vi "part_2.vi"() -> ()   [LabVIEW 2023]
panel:
  in  "check":bool
  in  "stop":bool
  in  "stop 2":bool
  out "Array":bool[](array[boolean])
  in  "Enum":enum16{"XOr", "Or", "And"}(ring)
  out "Boolean 24":bool
  out "Boolean 23":bool
  out "Boolean 22":bool
  out "Boolean 21":bool
  out "Boolean 20":bool
  out "Boolean 19":bool
  out "Boolean 18":bool
  out "Boolean 17":bool
  in  "Boolean 16":bool
  in  "Boolean 15":bool
  in  "Boolean 14":bool
  in  "Boolean 13":bool
  in  "Boolean 12":bool
  in  "Boolean 11":bool
  in  "Boolean 10":bool
  in  "Boolean 9":bool
  in  "Boolean 8":bool
  in  "Boolean 7":bool
  in  "Boolean 6":bool
  in  "Boolean 5":bool
  in  "Boolean 4":bool
  in  "Boolean 3":bool
  in  "Boolean 2":bool
  in  "Boolean":bool
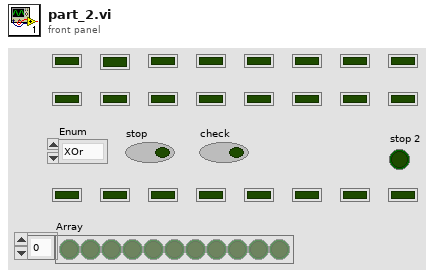
[diagram p1: front panel]
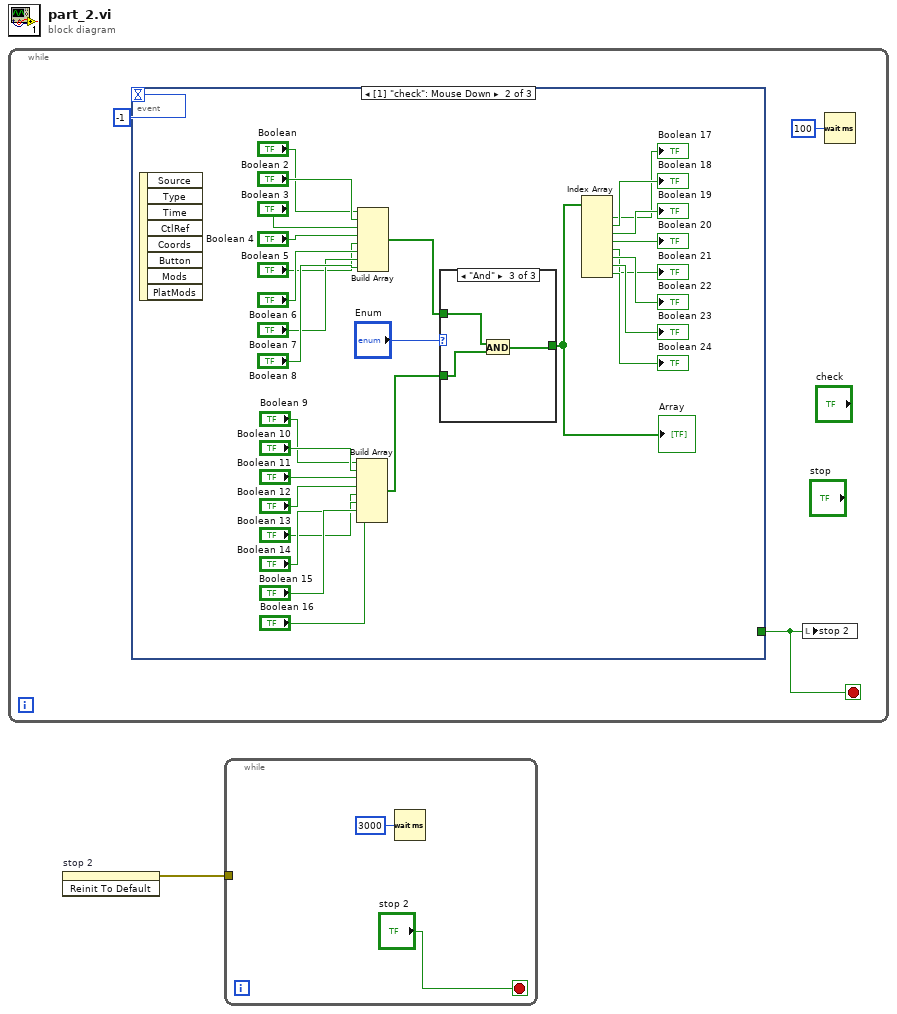
[diagram p0: block diagram]
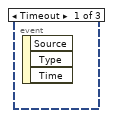
[diagram p2: hidden frame]
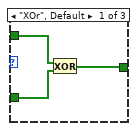
[diagram p3: hidden frame]
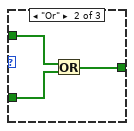
[diagram p4: hidden frame]
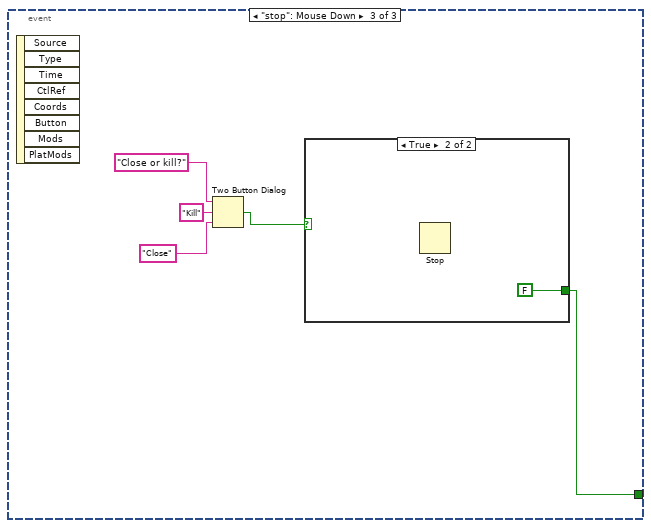
[diagram p5: hidden frame]
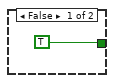
[diagram p6: hidden frame]
diagram:
  n1 = while {
    stop <- w3 stop-if-true
    n2 = event shown="[1] \"check\": Mouse Down" {
      selector: _ -> [_ _ _]
      dyn-events: _ -> [_ _ _]
      timeout: -1 -> [_ _ _]
      tunnel: [_ _ w42] -> w3
      event Timeout {
        n3 = event-data() -> ()  [unwired: 1 in, 3 out]
      }
      event "check": Mouse Down {
        n4 = event-data() -> ()  [unwired: 1 in, 8 out]
        n5 = Build Array("Boolean 9", "Boolean 10", "Boolean 11", "Boolean 12", "Boolean 13", "Boolean 14", "Boolean 15", "Boolean 16") -> (w23:bool[])
        n6 = Build Array("Boolean", "Boolean 2", "Boolean 3", "Boolean 4", "Boolean 5", "Boolean 6", "Boolean 7", "Boolean 8") -> (w22:bool[])
        n7 = case shown="\"And\"" "Enum" {
          tunnel: w22 -> [w33 w37 w40]
          tunnel: w23 -> [w34 w38 w41]
          tunnel: [w35 w36 w39] -> w24
          frame "XOr", Default {
            n8 = Exclusive Or(1:w34, 2:w33) -> (0:w35:bool[])
          }
          frame "Or" {
            n9 = Or(x=w37, y=w38) -> (x .or. y?=w36:bool[])
          }
          frame "And" {
            n10 = And(x=w40, y=w41) -> (x .and. y?=w39:bool[])
          }
        }
        "Array" <- w24
        n11 = Index Array(array=w24) -> (element #1=→"Boolean 17":bool, element #2=→"Boolean 18":bool, element #3=→"Boolean 19":bool, element #4=→"Boolean 20":bool, element #5=→"Boolean 21":bool, element #6=→"Boolean 22":bool, element #7=→"Boolean 23":bool, element #8=→"Boolean 24":bool)  [unwired: 8 in]
      }
      event "stop": Mouse Down {
        n12 = event-data() -> ()  [unwired: 1 in, 8 out]
        n13 = Two Button Dialog(message="Close or kill?", 1:"Close" ("F button name (\"Cancel\")"), 2:"Kill" ("T button name (\"OK\")")) -> (T button?=w46:bool)
        n14 = case shown="True" w46 {
          tunnel: [TRUE FALSE] -> w42
          frame False {
          }
          frame True {
            n15 = Stop() -> ()  [unwired: 1 in]
          }
        }
      }
    }
    n16 = local write "stop 2"(w3) -> ()
    n17 = Wait (ms)(milliseconds to wait=u32 100) -> ()  [unwired: 1 out]
  }
  n18 = invoke on="stop 2" class="Bool (strict)" method="Reinit To Default"() -> (error out=w1:errorcluster)  [unwired: 3 in, 2 out]
  n19 = while {
    tunnel: w1 -> [_]
    stop <- "stop 2" stop-if-true
    n20 = Wait (ms)(milliseconds to wait=u32 3000) -> ()  [unwired: 1 out]
  }
